vi "fake_inverse_josephus.vi"() -> ()   [LabVIEW 2019]
panel:
  out "Start at":dbl
  in  "Last":dbl
  in  "m":dbl
  in  "N":dbl
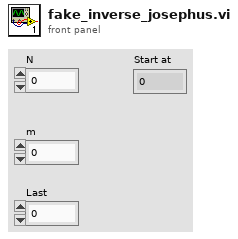
[diagram p1: front panel]
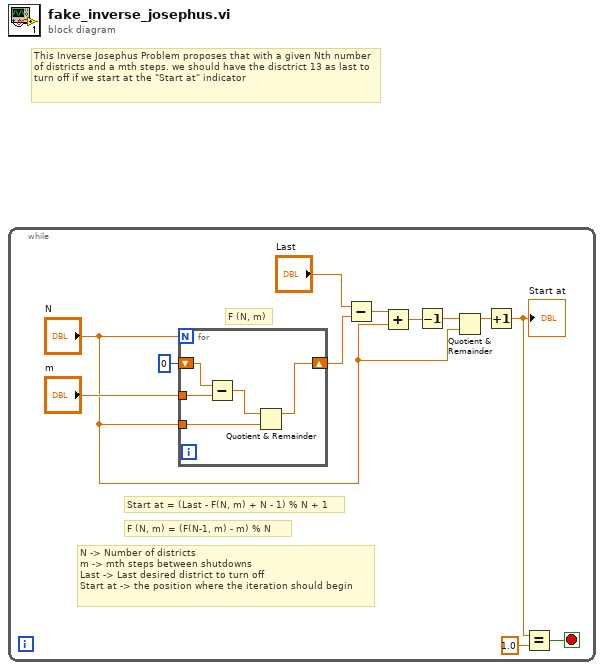
[diagram p0: block diagram]
diagram:
  # "This Inverse Josephus Problem proposes that with a given Nth number of districts and a mth steps. we should have the disctrict 13 as last to turn off if we start at the \"Start at\" indicator"
  n1 = while {
    stop <- w1 stop-if-true
    # "F (N, m) = (F(N-1, m) - m) % N"
    # "F (N, m)"
    # "Start at = (Last - F(N, m) + N - 1) % N + 1"
    # "N -> Number of districts\nm -> mth steps between shutdowns\nLast -> Last desired district to turn off\nStart at -> the position where the iteration should begin"
    n2 = for {
      N: "N" -> [_]
      shift-right: [w13] -> w9
      shift-left: 0 -> [w14]
      tunnel: "N" -> [w16]
      tunnel: "m" -> [w15]
      n3 = Subtract(x=w14, y=w15) -> (x-y=w17:dbl)
      n4 = Quotient & Remainder(x=w17, y=w16) -> (x-y*floor(x/y)=w13:dbl)  [unwired: 1 out]
    }
    n5 = Subtract(x="Last", y=w9) -> (x-y=w8:dbl)
    n6 = Add(x=w8, y="N") -> (x+y=w7:dbl)
    n7 = Decrement(x=w7) -> (x-1=w6:dbl)
    n8 = Quotient & Remainder(x=w6, y="N") -> (x-y*floor(x/y)=w5:dbl)  [unwired: 1 out]
    n9 = Increment(x=w5) -> (x+1=w2:dbl)
    "Start at" <- w2
    n10 = Equal?(x=w2, y=1.0) -> (x = y?=w1:bool)
  }
